vi "Drive Teleop.vi"(6 "Auto Align":bool, 8 "Fast Mode":bool, 9 "Quick turn":bool, 10 "Turn":dbl, 11 "Forward":dbl) -> ()   [LabVIEW 2018]
uses:
  <vilib>/Rock Robotics/Network Tables/NT Read Number.vi
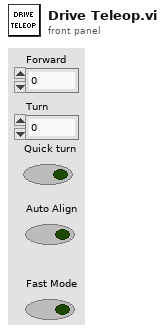
[diagram p1: front panel]
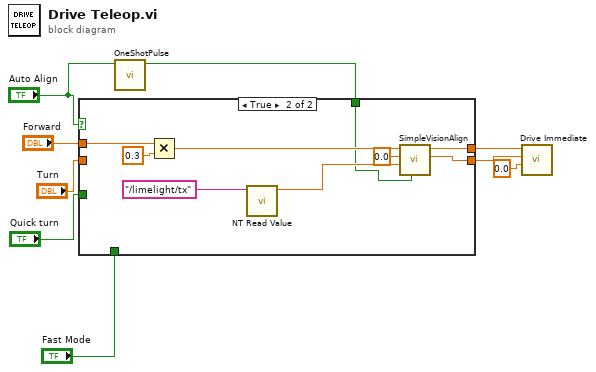
[diagram p0: block diagram]
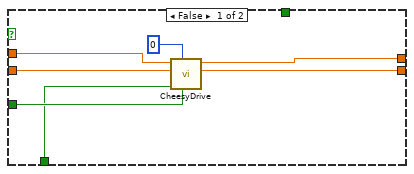
[diagram p2: hidden frame]
diagram:
  n1 = call "OneShotPulse.vi"("Input"="Auto Align") -> ("Output"=w1:bool)  [unwired: 10 in]
  n2 = case shown="True" "Auto Align" {
    tunnel: "Quick turn" -> [w16 _]
    tunnel: "Turn" -> [w11 _]
    tunnel: "Forward" -> [w12 w24]
    tunnel: [w14 w21] -> w5
    tunnel: [w13 w20] -> w4
    tunnel: "Fast Mode" -> [w10 _]
    tunnel: w1 -> [_ w17]
    frame False {
      n3 = call "CheesyDrive.vi"("Quickturn"=w16, "SlowMode"=u32 0, "Fast Mode"=w10, "Wheel"=w11, "Throttle"=w12) -> ("Right PWM"=w13:dbl, "Left PWM"=w14:dbl)  [unwired: 5 in]
    }
    frame True {
      n4 = Multiply(x=w24, y=0.3) -> (x*y=w25:dbl)
      n5 = call-poly <vilib>:"NT Read Value.vi"("Name"="/limelight/tx") -> ("Numeric"=w22:dbl)  [unwired: 9 in, 1 out]
      n6 = call "SimpleVisionAlign.vi"("Reset"=w17, "Target Offset"=w22, "Gyro"=0.0, "Throttle"=w25) -> ("Right Power"=w20:dbl, "Left Power"=w21:dbl)  [unwired: 6 in]
    }
  }
  n7 = call "Drive Immediate.vi"("Deadband Value"=0.0, "Right Setpoint"=w4, "Left Setpoint"=w5) -> ()  [unwired: 8 in, 1 out]
